vi "Read Strings[].vi"(8 "error in (no error)":errorcluster, 11 "BreadcrumbNavigation in":refnum<class "BreadcrumbNavigator.lvclass">) -> (0 "error out":errorcluster, 2 "Strings[]":string[](array[string]), 3 "BreadcrumbNavigation out":refnum<class "BreadcrumbNavigator.lvclass">)   [LabVIEW 2015, in "BreadcrumbNavigator.lvclass"]
uses:
  BreadcrumbNavigator.lvclass
  BreadcrumbNavigator.lvclass/BreadcrumbNavigator.ctl
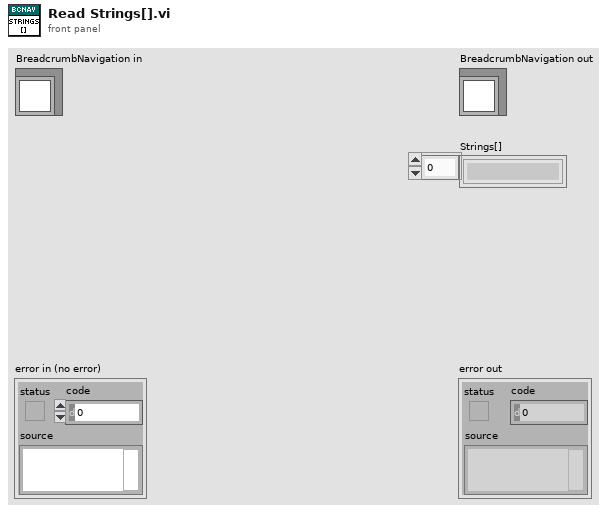
[diagram p1: front panel]
types:
  T1 = typedef "BreadcrumbNavigation.lvclass/State Data.ctl" = cluster{"Strings[]":string[], "CurrentLeftMostItem":i32, "Delimeter":string}
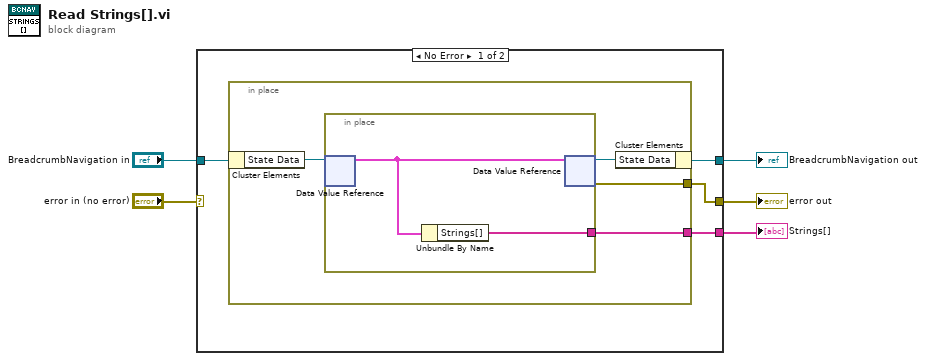
[diagram p0: block diagram]
diagram:
  n1 = case shown="No Error" "error in (no error)" {
    selector: "error in (no error)" -> [_ w17]
    tunnel: [w8 w17] -> w4
    tunnel: [w7 w16] -> w2
    tunnel: "BreadcrumbNavigation in" -> [w9 w16]
    tunnel: [w6 _] -> w1
    frame No Error {
      n2 = in-place {
        in-place-border: [w12] -> w8
        in-place-border: [w10] -> w6
        n3 = in-place-cluster #1(w9) -> ("State Data"=w13:refnum<data-value>)
        n4 = in-place {
          in-place-border: [w14] -> w10
          n5 = in-place-dvr #2(w13) -> (w15:T1)  [unwired: 1 out]
          n6 = Unbundle By Name(w15) -> ("Strings[]"=w14:string[])
          n7 = in-place-dvr #2(w15) -> (w11:refnum<data-value>, w12:errorcluster)
        }
        n8 = in-place-cluster #1("State Data"=w11) -> (w7:refnum<class "BreadcrumbNavigator.lvclass">)
      }
    }
    frame Error {
    }
  }
  "error out" <- w4
  "BreadcrumbNavigation out" <- w2
  "Strings[]" <- w1
